vi "MEScope_RUNSILOTEST.vi"(8 "error in (no error)":errorcluster) -> (0 "error out":errorcluster, 1 "return type":i32, 3 "pnTestResult":i32)   [LabVIEW 2015]
doc: "MEScope_RunSiloTest \nDescription:\nThis function will command the DSP to run its Silo memory test.\nDetail:\nint MEScope_RunSiloTest (\nint *pnTestResult\n);\n\nParameters:\nint *pnTestResult- pointer to an integer, filled with the result of the test. \n\nPASSED = 1\nFAILED = 0\n\nReturn Values:\nThis function returns a 0 if the function completed successfully. A non-zero return code will indicate error. \nRemarks:\nThis functions tests the 512K words of external static RAM.\nThe RAM is organized as 16 pages of 32 K words each. The memory in each page starts at address 0x8000 and extends up to 0xFFFF. \nOnly odd numbered pages are populated, starting with page 1 and extending up to page 0x1F (31)."
uses:
  ScannerDiagDLL.dll
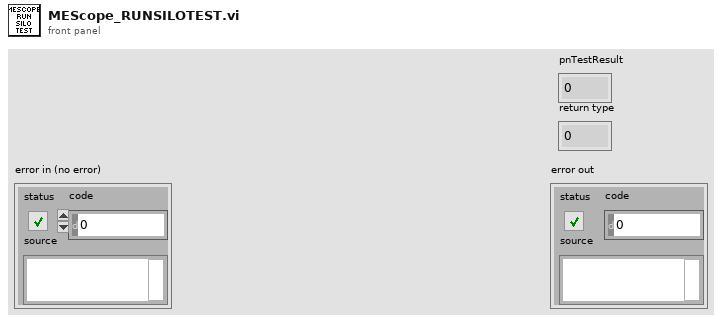
[diagram p1: front panel]
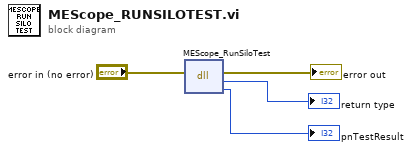
[diagram p0: block diagram]
diagram:
  n1 = dll-call lib="C:/ModisEdge/Scope/Test Sequence/Code Modules/DLL/ScannerDiagDLL.dll" fn="MEScope_RunSiloTest"(error in="error in (no error)") -> (error out=→"error out":errorcluster, "return type"=→"return type":i32, "pnTestResult"=→"pnTestResult":i32)  [unwired: 3 in, 1 out]
